vi "autosave_test.vi"() -> ()   [LabVIEW 2018]
uses:
  <vilib>/ErrorRing/Error Ring.xnode
panel:
  out "x-y":dbl
  out "StartTime":timestamp
  out "date/time string":string
  in  "¸ê®Æ§¨\nµù°O>":string
  out "triggered 2":dynamicdata(graph)
  out "Numeric":i32
  out "size(s)":i32
  out "low":bool
  out "da":bool
  out "on":bool
  out "raw 2":dynamicdata(graph)
  in  "Stop":bool
  out "triggered":dynamicdata(graph)
  out "raw":dynamicdata(graph)
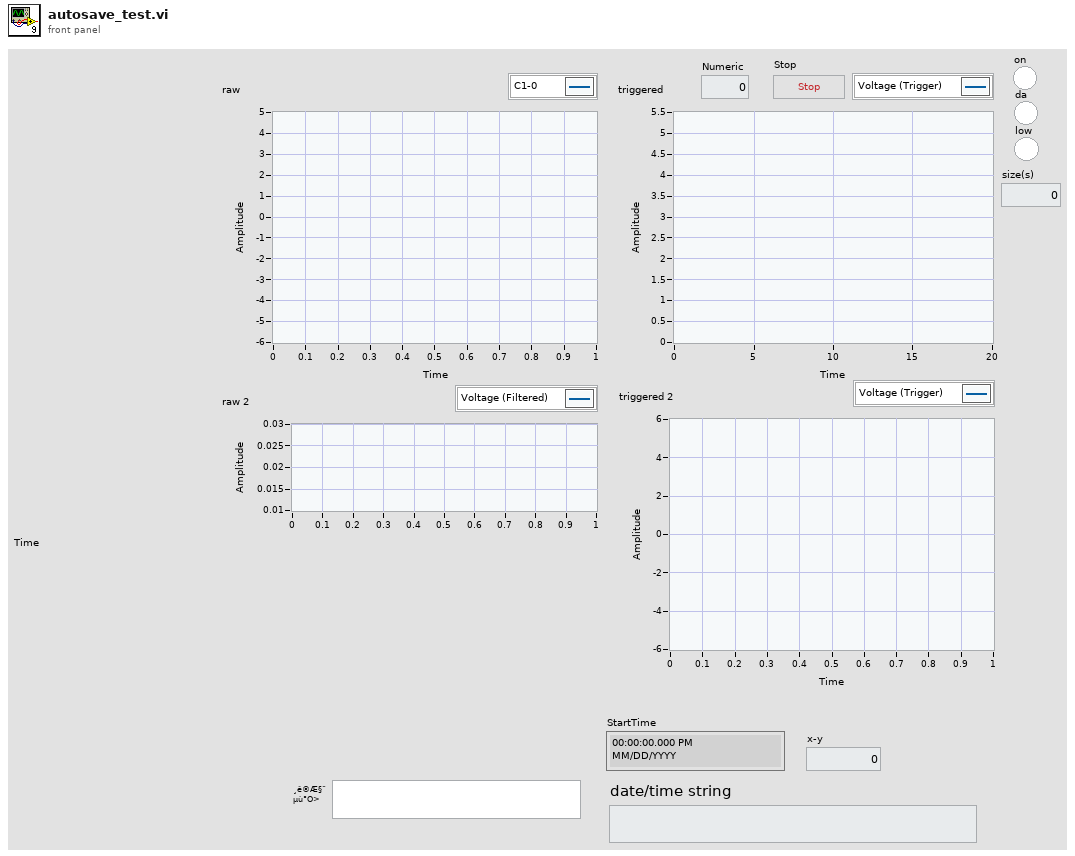
[diagram p1: front panel]
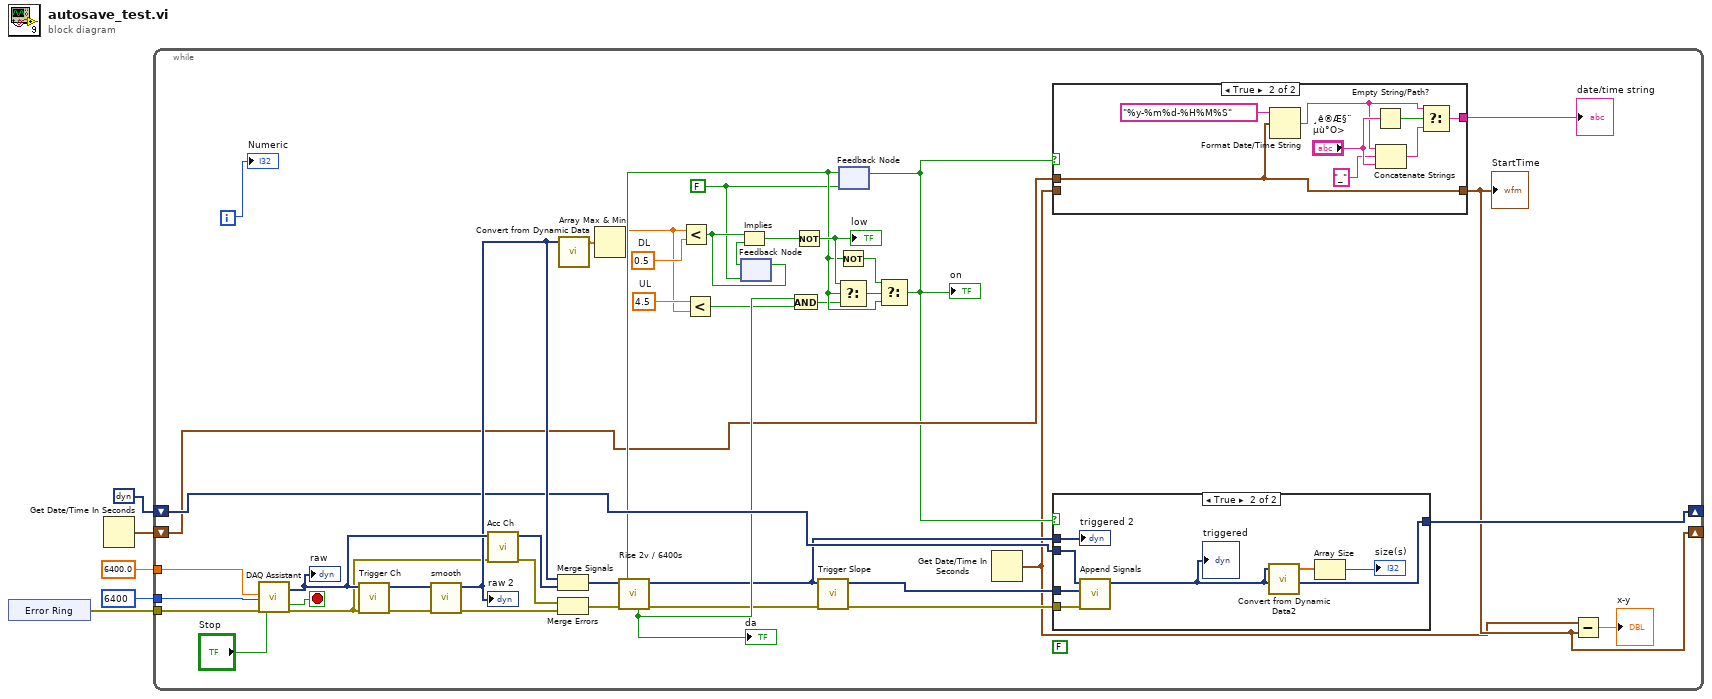
[diagram p0: block diagram]
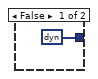
[diagram p3: hidden frame]
diagram:
  n1 = xnode "Error Ring"() -> ("error out"=w5:errorcluster)
  n2 = Get Date/Time In Seconds() -> (seconds since 1Jan1904=w1:timestamp)
  n3 = while {
    tunnel: w5 -> [w48]
    tunnel: 6400.0 ("rate") -> [w47]
    tunnel: 6400 ("number of samples") -> [w46]
    shift-right: [w33] -> _
    shift-left: dynamicdata [] ("Waveform Graph") -> [w34]
    shift-right: [w9] -> _
    shift-left: w1 -> [w12]
    i -> [w25]
    stop <- w44 stop-if-true
    w6 = FALSE
    w22 = 4.5  # UL
    (unwired) FALSE
    w38 = 0.5  # DL
    n4 = call "DAQ Assistant"("rate"=w47, "number of samples"=w46, "error in"=w48, "stop (F)"="Stop") -> ("data"=w42:dynamicdata, "stopped"=w44:bool, "error out"=w19:errorcluster)  [unwired: 12 in, 1 out]
    "raw" <- w42
    n5 = call "Trigger Ch"("error in (no error)"=w19, "Signals"=w42) -> ("error out"=w18:errorcluster, "Signal Out"=w43:dynamicdata)  [unwired: 8 in]
    n6 = call "smooth"("error in (no error)"=w18, "Signal"=w43) -> ("error out"=w17:errorcluster, "Filtered Signal"=w39:dynamicdata)  [unwired: 8 in]
    "raw 2" <- w39
    n7 = call "Acc Ch"("error in (no error)"=w19, "Signals"=w42) -> ("error out"=w15:errorcluster, "Signal Out"=w41:dynamicdata)  [unwired: 8 in]
    n8 = Merge Signals(w39, w41) -> (w31:dynamicdata)
    n9 = Merge Errors(w15, w17) -> (w16:errorcluster)
    n10 = call "Convert from Dynamic Data"("Dynamic Data Type"=w39) -> ("Array"=w32:dbl[])  [unwired: 3 in]
    n11 = Array Max & Min(array=w32) -> (max value=w21:dbl)  [unwired: 3 out]
    n12 = Less?(x=w21, y=w38) -> (x < y?=w35:bool)
    n13 = Less?(x=w22, y=w21) -> (x < y?=w20:bool)
    n14 = feedback-in #1(w35) -> ()
    n15 = feedback #1(w6) -> (w36:bool)
    n16 = Implies(1:w36, 2:w35) -> (0:w37:bool)
    n17 = Not(x=w37) -> (.not. x?=w28:bool)
    "low" <- w28
    n18 = feedback #2(w6) -> (w27:bool)
    n19 = call "Rise 2v / 6400s"("Manual Trigger"=w27, "error in (no error)"=w16, "Signals"=w31) -> ("error out"=w14:errorcluster, "Triggered Signals"=w24:dynamicdata, "Data Available"=w29:bool)  [unwired: 5 in, 1 out]
    "da" <- w29
    n20 = And(x=w29, y=w20) -> (x .and. y?=w23:bool)
    n21 = call "Trigger Slope"("error in (no error)"=w14, "Signals"=w24) -> ("error out"=w13:errorcluster, "Signal Out"=w26:dynamicdata)  [unwired: 8 in]
    n22 = Not(x=w27) -> (.not. x?=w40:bool)
    n23 = Select(t=w28, s=w27, f=w23) -> (s? t:f=w30:bool)
    n24 = Select(t=w40, s=w30, f=w27) -> (s? t:f=w11:bool)
    "on" <- w11
    n25 = feedback-in #2(w11) -> ()
    n26 = Get Date/Time In Seconds() -> (seconds since 1Jan1904=w8:timestamp)
    n27 = case shown="True" w11 {
      tunnel: [w49 w52] -> w9
      tunnel: w12 -> [_ w52]
      tunnel: [_ w51] -> w10
      tunnel: w8 -> [w49 _]
      frame False {
      }
      frame True {
        n28 = Format Date/Time String(time format string (%c)="%y-%m%d-%H%M%S", seconds (now)=w52) -> (date/time string=w50:string)  [unwired: 1 in]
        n29 = Empty String/Path?(string/path="¸ê®Æ§¨\nµù°O>") -> (empty?=w56:bool)
        n30 = Concatenate Strings(w50, "_" ("string"), "¸ê®Æ§¨\nµù°O>") -> (w55:string)
        n31 = Select(t=w50, s=w56, f=w55) -> (s? t:f=w51:string)
      }
    }
    "date/time string" <- w10
    "StartTime" <- w9
    n32 = case shown="True" w11 {
      tunnel: w34 -> [_ w65]
      tunnel: [dynamicdata [] ("Waveform Graph") w63] -> w33
      tunnel: w26 -> [_ w64]
      tunnel: w24 -> [_ w60]
      tunnel: w13 -> [_ w59]
      frame False {
      }
      frame True {
        n33 = call "Append Signals"("error in (no error)"=w59, "Input Signal B"=w64, "Input Signal A"=w65) -> ("Appended Signals"=w63:dynamicdata)  [unwired: 7 in, 1 out]
        "triggered" <- w63
        n34 = call "Convert from Dynamic Data2"("Dynamic Data Type"=w63) -> ("Array"=w62:dbl[])  [unwired: 3 in]
        n35 = Array Size(array=w62) -> (size(s)=→"size(s)":i32)
        "triggered 2" <- w60
      }
    }
    n36 = Subtract(x=w8, y=w9) -> (x-y=→"x-y":dbl)
    "Numeric" <- w25
  }
